vi "1_Frekans.vi"(10 "Ölçüm Süresi [sn]":i32=60, 11 "Remote IP Address":string="10.1.21.100") -> (0 "error out":errorcluster, 2 "Frekans":sgl[][](array[numeric]))   [LabVIEW 2014]
panel:
  out "Frekans FD2 f":sgl[](array[numeric]) format="%_6f"
  out "Frekans FD1 f":sgl[](array[numeric]) format="%_6f"
  in  "Frekans FD2 f Register":u16=685
  out "Numeric":i32
  in  "Frekans FD1 f Register":u16=21
  out "time stamp":timestamp=timestamp(1426515300 s since 1904-01-01) format="%<%H:%M:%S>T"
  in  "Remote Port":u16=1502
  in  "Stop":bool
  # "MB Ethernet Example Master.vi\n\nInstructions\n1. Run MB Ethernet Example Slave.vi\n2. Run this VI.\n3. Modify the discrete inputs or input registers on the slave -> they're updated on the master.\n4. Modify the coils and registers on the master -> they're updated on the slave."
  # "TCP Parameters"
  # "Slave Read-only Registers"
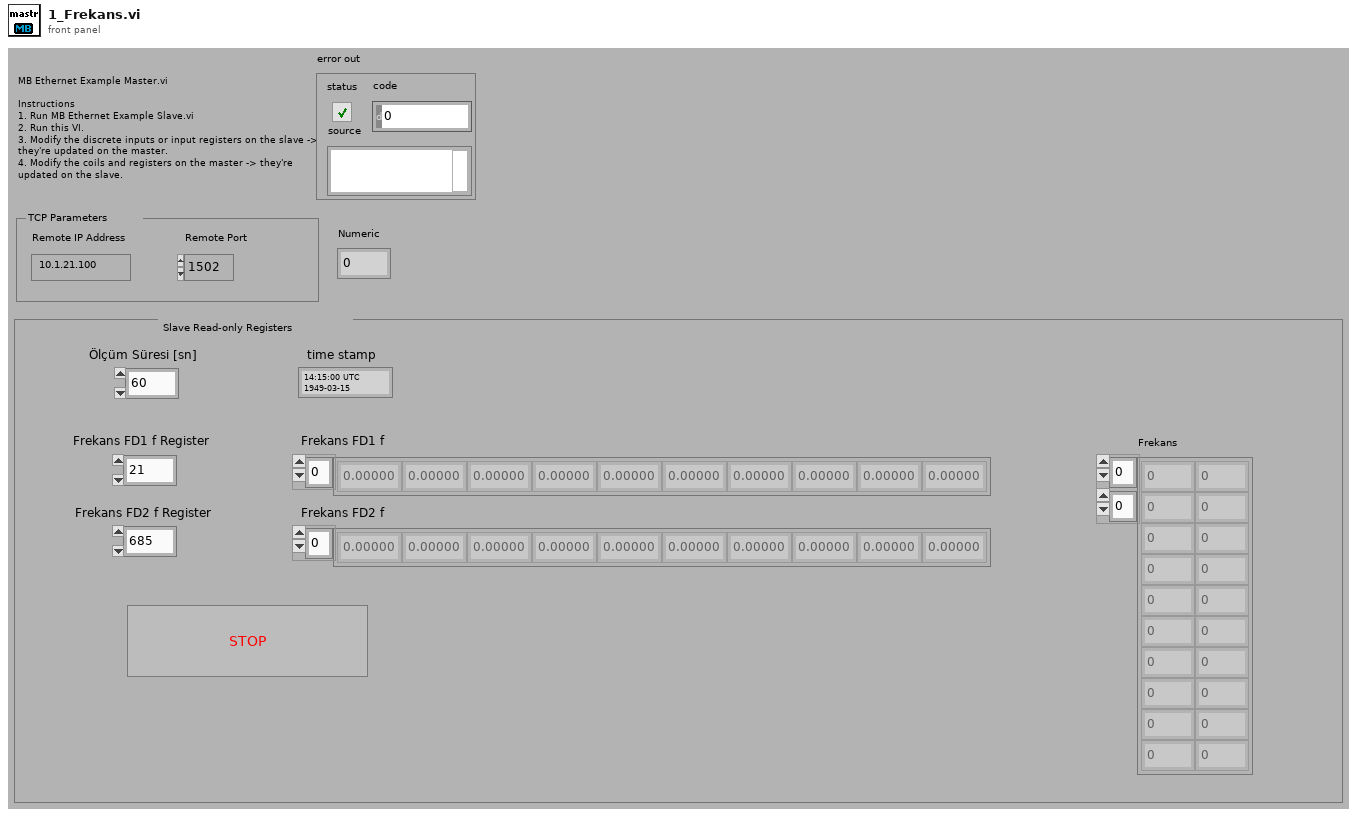
[diagram p1: front panel]
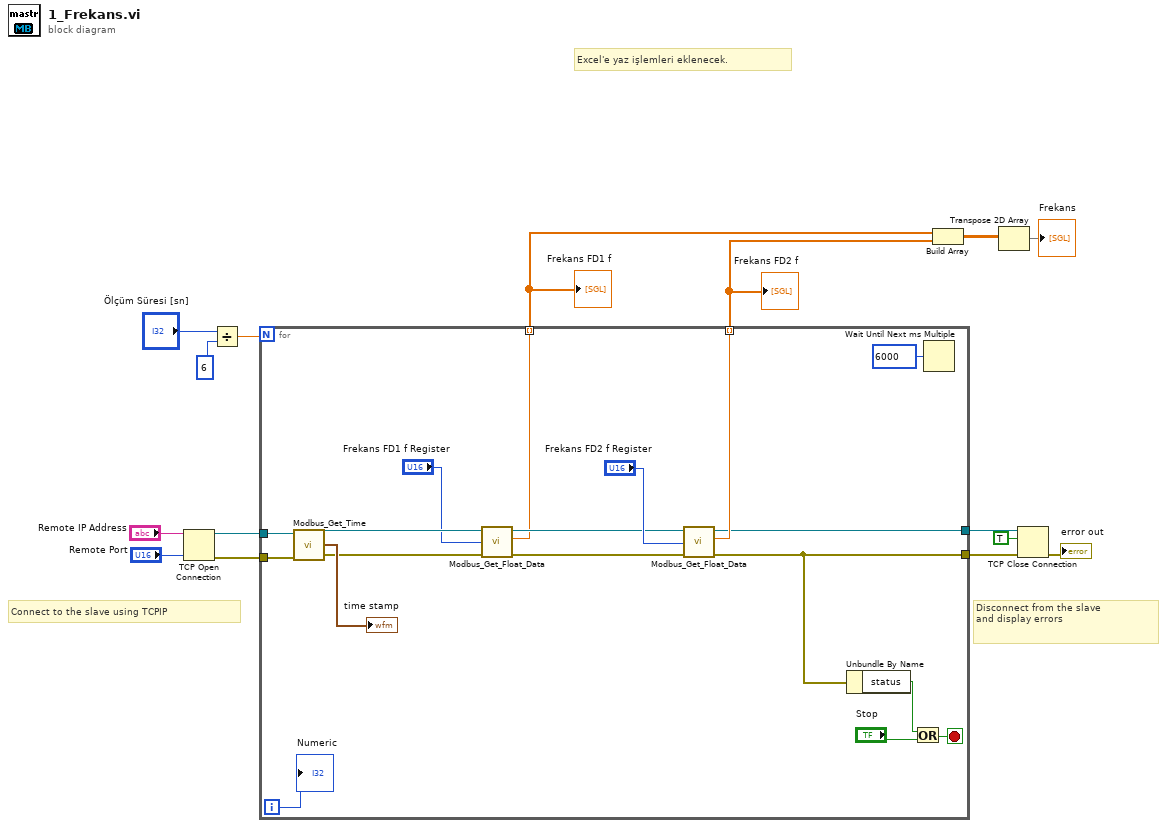
[diagram p0: block diagram]
diagram:
  # "Excel'e yaz işlemleri eklenecek."
  # "Disconnect from the slave\nand display errors"
  # "Connect to the slave using TCPIP"
  n1 = TCP Open Connection(address="Remote IP Address", remote port or service name="Remote Port") -> (connection ID=w13:refnum<k5>, error out=w12:errorcluster)  [unwired: 1 in, 2 out]
  n2 = Divide(x="Ölçüm Süresi [sn]", y=6) -> (x/y=w8:dbl)
  n3 = for {
    N: w8 -> [_]
    tunnel: [w18] -> w11
    tunnel: w13 -> [w31]
    tunnel: w12 -> [w30]
    tunnel: [w17] -> w5
    tunnel: [w20] -> w3 mode=indexing
    tunnel: [w19] -> w4 mode=indexing
    i -> [w25]
    stop <- w16 stop-if-true
    n4 = call "Modbus_Get_Time.vi"("error in (no error)"=w30, "TCP Network Connection in"=w31) -> ("error out"=w26:errorcluster, "Time Stamp"=→"time stamp":timestamp, "TCP Network Connection out"=w28:refnum<k5>)  [unwired: 6 in, 1 out]
    n5 = call "Modbus_Get_Float_Data.vi"("error in (no error)"=w26, "Starting Address (2 Bytes)"="Frekans FD1 f Register", "TCP Network Connection in"=w28) -> ("error out"=w22:errorcluster, "Numeric"=w20:sgl, "TCP Network Connection out"=w21:refnum<k5>)  [unwired: 5 in, 1 out]
    n6 = call "Modbus_Get_Float_Data.vi"("error in (no error)"=w22, "Starting Address (2 Bytes)"="Frekans FD2 f Register", "TCP Network Connection in"=w21) -> ("error out"=w18:errorcluster, "Numeric"=w19:sgl, "TCP Network Connection out"=w17:refnum<k5>)  [unwired: 5 in, 1 out]
    n7 = Unbundle By Name(w18) -> ("status"=w32:bool)
    n8 = Or(x=w32, y="Stop") -> (x .or. y?=w16:bool)
    n9 = Wait Until Next ms Multiple(millisecond multiple=u32 6000) -> ()  [unwired: 1 out]
    "Numeric" <- w25
  }
  "Frekans FD1 f" <- w3
  "Frekans FD2 f" <- w4
  n10 = Build Array(w3, w4) -> (w2:sgl[][])
  n11 = Transpose 2D Array(2D array=w2) -> (transposed array=→"Frekans":sgl[][])
  n12 = TCP Close Connection(connection ID=w5, abort (F)=TRUE, error in (no error)=w11) -> (error out=→"error out":errorcluster)  [unwired: 1 out]
